vi "Handle Messages.vi"(8 "error in (no error)":errorcluster, 9 "Message Data":variant, 10 "Message":string, 11 "Device Under Test In":refnum<class "Device Under Test.lvclass">) -> (0 "error out":errorcluster, 3 "Device Under Test Out":refnum<class "Device Under Test.lvclass">)   [LabVIEW 2020, in "Device Under Test.lvclass"]
uses:
  Device Under Test.lvclass
  C:/Program Files (x86)/National Instruments/LabVIEW 2020/vi.lib/Astemes/Triarc Framework/Process/Process.lvclass
  Device Under Test.lvclass/Device Under Test.ctl
  Private/Self Test Reply Payload.ctl
  <vilib>/Astemes/Triarc Framework/Process/Process.lvclass/Process.ctl
  <vilib>/Astemes/Triarc Framework/Process/Private/SubVIs/Handle Debug Data.vi
  <vilib>/Utility/error.llb/Error Cluster From Error Code.vi
  <vilib>/Astemes/Triarc Framework/Process/Public/Lifecycle/Get Lifecycle State.vi
  <vilib>/Astemes/Triarc Framework/View/View.lvclass
  <vilib>/Astemes/Triarc Framework/Callback/Callback.lvclass
  <vilib>/Astemes/Triarc Framework/Process/Process.lvclass
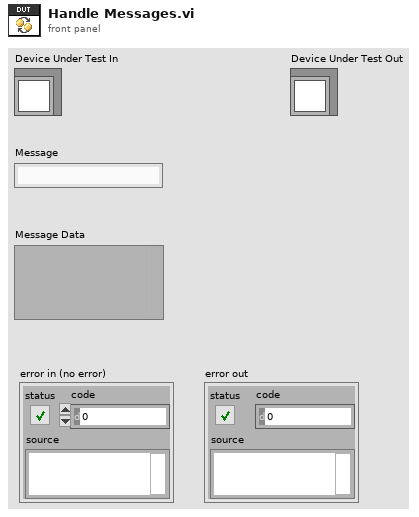
[diagram p1: front panel]
types:
  T1 = typedef "Device Under Test.lvclass/Self Test Reply Payload.ctl" = cluster{"Result":bool, "Self Test Error":errorcluster}
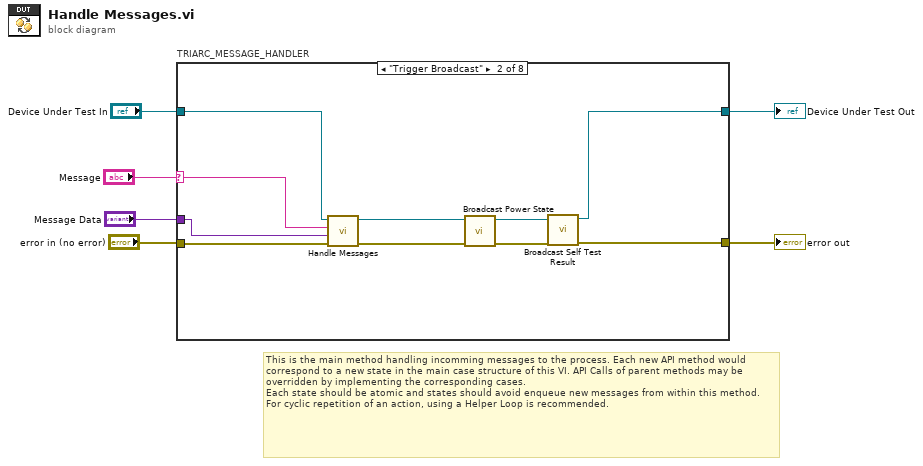
[diagram p0: block diagram]
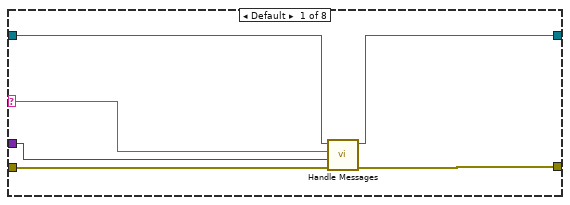
[diagram p2: hidden frame]
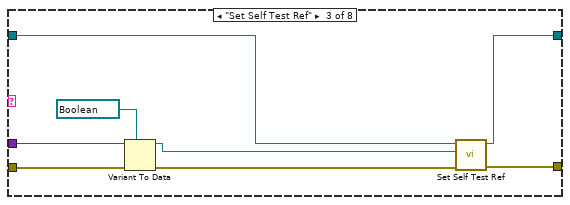
[diagram p3: hidden frame]
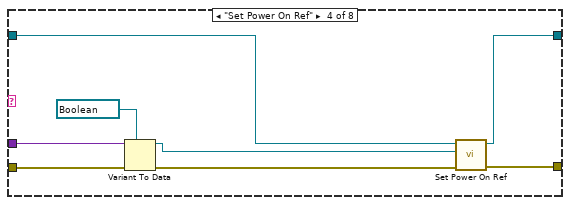
[diagram p4: hidden frame]
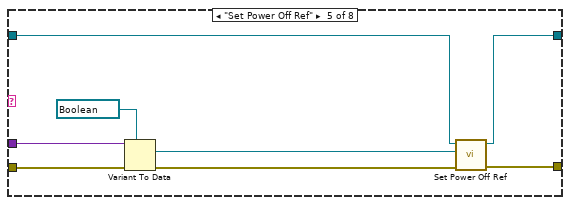
[diagram p5: hidden frame]
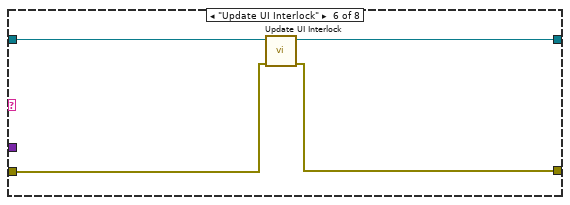
[diagram p6: hidden frame]
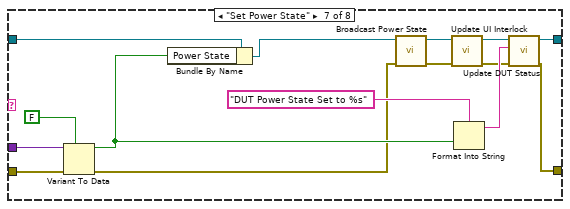
[diagram p7: hidden frame]
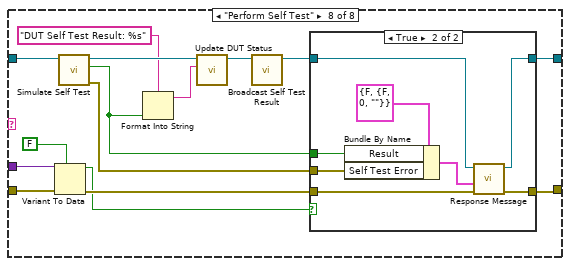
[diagram p8: hidden frame]
diagram:
  # "This is the main method handling incomming messages to the process. Each new API method would correspond to a new state in the main case structure of this VI. API Calls of parent methods may be overridden by implementing the corresponding cases.\nEach state should be atomic and states should avoid enqueue new messages from within this method. For cyclic repetition of an action, using a Helper Loop is recommended."
  n1 = case "TRIARC_MESSAGE_HANDLER" shown="\"Trigger Broadcast\"" "Message" {
    selector: "Message" -> [w10 w20 _ _ _ _ _ _]
    tunnel: "error in (no error)" -> [w9 w19 w30 w38 w46 w49 w63 w70]
    tunnel: "Device Under Test In" -> [w12 w22 w23 w31 w44 w50 w58 w69]
    tunnel: "Message Data" -> [w11 w21 w29 w37 w45 _ w64 w66]
    tunnel: [w8 w13 w25 w34 w40 w47 w59 w67] -> w2
    tunnel: [w7 w15 w28 w36 w43 w48 w60 w68] -> w1
    frame Default {
      n2 = call-parent "Handle Messages.vi"("error in (no error)"=w9, "Message Data"=w11, "Message"=w10, "View In"=w12) -> ("error out"=w8:errorcluster, "View Out"=w7:refnum<class "Device Under Test.lvclass">)  [unwired: 6 in]
    }
    frame "Trigger Broadcast" {
      n3 = call-parent "Handle Messages.vi"("error in (no error)"=w19, "Message Data"=w21, "Message"=w20, "View In"=w22) -> ("error out"=w14:errorcluster, "View Out"=w16:refnum<class "Device Under Test.lvclass">)  [unwired: 6 in]
      n4 = call "Broadcast Power State.vi"("error in (no error)"=w14, "Device Under Test in"=w16) -> ("error out"=w17:errorcluster, "Device Under Test out"=w18:refnum<class "Device Under Test.lvclass">)  [unwired: 8 in]
      n5 = call "Broadcast Self Test Result.vi"("error in (no error)"=w17, "Device Under Test in"=w18) -> ("error out"=w13:errorcluster, "Device Under Test out"=w15:refnum<class "Device Under Test.lvclass">)  [unwired: 8 in]
    }
    frame "Set Self Test Ref" {
      n6 = Variant To Data(error in=w30, type=refnum<vi> refnum ("data"), Variant=w29) -> (data=w27:refnum<vi>, error out=w24:errorcluster)
      n7 = call "Set Self Test Ref.vi"("error in (no error)"=w24, "Self Test"=w27, "Device Under Test In"=w23) -> ("error out"=w25:errorcluster, "Device Under Test Out"=w28:refnum<class "Device Under Test.lvclass">)  [unwired: 7 in]
    }
    frame "Set Power On Ref" {
      n8 = Variant To Data(error in=w38, type=refnum<vi> refnum ("data"), Variant=w37) -> (data=w32:refnum<vi>, error out=w33:errorcluster)
      n9 = call "Set Power On Ref.vi"("error in (no error)"=w33, "Self Test"=w32, "Device Under Test In"=w31) -> ("error out"=w34:errorcluster, "Device Under Test Out"=w36:refnum<class "Device Under Test.lvclass">)  [unwired: 7 in]
    }
    frame "Set Power Off Ref" {
      n10 = Variant To Data(error in=w46, type=refnum<vi> refnum ("data"), Variant=w45) -> (data=w42:refnum<vi>, error out=w39:errorcluster)
      n11 = call "Set Power Off Ref.vi"("error in (no error)"=w39, "Self Test"=w42, "Device Under Test In"=w44) -> ("error out"=w40:errorcluster, "Device Under Test Out"=w43:refnum<class "Device Under Test.lvclass">)  [unwired: 7 in]
    }
    frame "Update UI Interlock" {
      n12 = call "Update UI Interlock.vi"("error in (no error)"=w49, "Device Under Test In"=w50) -> ("error out"=w47:errorcluster, "Device Under Test Out"=w48:refnum<class "Device Under Test.lvclass">)  [unwired: 8 in]
    }
    frame "Set Power State" {
      n13 = Variant To Data(error in=w63, type=FALSE ("Boolean"), Variant=w64) -> (data=w57:bool, error out=w55:errorcluster)
      n14 = Bundle By Name(cluster=w58, "Power State"=w57) -> (w56:refnum<class "Device Under Test.lvclass">)
      n15 = call "Broadcast Power State.vi"("error in (no error)"=w55, "Device Under Test in"=w56) -> ("error out"=w54:errorcluster, "Device Under Test out"=w52:refnum<class "Device Under Test.lvclass">)  [unwired: 8 in]
      n16 = call "Update UI Interlock.vi"("error in (no error)"=w54, "Device Under Test In"=w52) -> ("error out"=w53:errorcluster, "Device Under Test Out"=w51:refnum<class "Device Under Test.lvclass">)  [unwired: 8 in]
      n17 = Format Into String(format string="DUT Power State Set to %s", w57) -> (resulting string=w62:string)  [unwired: 2 in, 1 out]
      n18 = call "Update DUT Status.vi"("error in (no error)"=w53, "String"=w62, "Device Under Test In"=w51) -> ("error out"=w59:errorcluster, "Device Under Test Out"=w60:refnum<class "Device Under Test.lvclass">)  [unwired: 7 in]
    }
    frame "Perform Self Test" {
      n19 = Variant To Data(error in=w70, type=FALSE, Variant=w66) -> (data=w77:bool, error out=w78:errorcluster)
      n20 = call "Simulate Self Test.vi"("Device Under Test In"=w69) -> ("error out"=w79:errorcluster, "Pass"=w71:bool, "Device Under Test Out"=w76:refnum<class "Device Under Test.lvclass">)  [unwired: 8 in]
      n21 = Format Into String(format string="DUT Self Test Result: %s", w71) -> (resulting string=w74:string)  [unwired: 2 in, 1 out]
      n22 = call "Update DUT Status.vi"("String"=w74, "Device Under Test In"=w76) -> ("Device Under Test Out"=w72:refnum<class "Device Under Test.lvclass">)  [unwired: 8 in, 1 out]
      n23 = call "Broadcast Self Test Result.vi"("Device Under Test in"=w72) -> ("Device Under Test out"=w73:refnum<class "Device Under Test.lvclass">)  [unwired: 9 in, 1 out]
      n24 = case shown="True" w77 {
        tunnel: [w82 w90] -> w68
        tunnel: w73 -> [w82 w89]
        tunnel: w71 -> [_ w87]
        tunnel: w79 -> [_ w86]
        tunnel: w78 -> [w81 w84]
        tunnel: [w81 w83] -> w67
        frame False {
        }
        frame True {
          n25 = Bundle By Name(cluster=T1 {"Result"=FALSE, "Self Test Error"={"status"=FALSE, "code"=0, "source"=""}} ("Perform Self Test (Reply Payload)"), "Result"=w87, "Self Test Error"=w86) -> (w85:T1)
          n26 = call <vilib>:"Response Message.vi"("error in (no error)"=w84, "Response Message Data"=w85, "Process In"=w89) -> ("error out"=w83:errorcluster, "Process Out"=w90:refnum<class "Device Under Test.lvclass">)  [unwired: 7 in]
        }
      }
    }
  }
  "error out" <- w2
  "Device Under Test Out" <- w1
